vi "Determine Archive File Types.vi"(1 "2 LBCB Archiving Mode":bool, 2 "Number of\nLBCBs In":T1) -> (0 "File Type Indexes":i32[](array[numeric]))   [LabVIEW 2009]
uses:
  Data Access Objects/Application/Number Of LBCBs.ctl
panel:
  in  "File Type Index Matrix":i32[][](array[numeric])=[[0, 0, 0], [2, 1, 1], [4, 2, 2], [7, 4, 3], [-1, 5, 6], [-1, 7, 9], [-1, 8, -1], [-1, -1, -1]]
  # "1 LBCB"
  # "2\nLBCBs"
  # "Combined"
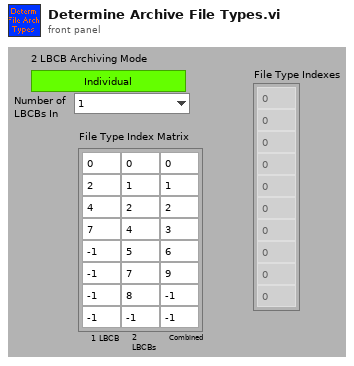
[diagram p1: front panel]
types:
  T1 = typedef "Number Of LBCBs.ctl" = enum16{"1", "2"}
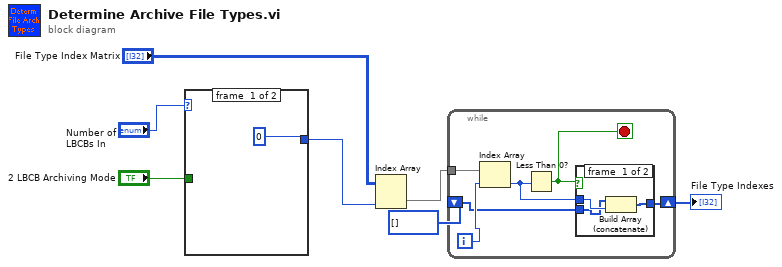
[diagram p0: block diagram]
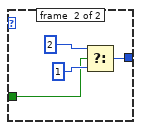
[diagram p3: hidden frame]
diagram:
  n1 = case shown="\"2\"" "Number of\nLBCBs In" {
    tunnel: [0 w12] -> w7
    tunnel: "2 LBCB Archiving Mode" -> [_ w9]
    frame #0 {
    }
    frame #1 {
      n2 = Select(t=2, s=w9, f=1) -> (s? t:f=w12:i32)
    }
  }
  n3 = Index Array(array="File Type Index Matrix", index (col)=w7) -> (element=w3:i32[])  [unwired: 1 in]
  n4 = while {
    tunnel: w3 -> [w18]
    shift-right: [w15] -> w2
    shift-left: i32[] [] -> [w13]
    i -> [w17]
    stop <- w14 stop-if-true
    n5 = Index Array(array=w18, index=w17) -> (element=w16:i32)
    n6 = Less Than 0?(x=w16) -> (x < 0?=w14:bool)
    n7 = case shown="False" w14 {
      tunnel: w16 -> [w20 _]
      tunnel: [w21 w22] -> w15
      tunnel: w13 -> [w19 w22]
      frame #0 {
        n8 = Build Array (concatenate)(w19, w20) -> (w21:i32[])
      }
      frame #1 {
      }
    }
  }
  "File Type Indexes" <- w2
